vi "Initialize.vi"(8 "error in (no error)":errorcluster, 11 "UDP Thread UI in":refnum<class "UDP Thread User Interface.lvclass">) -> (0 "error out":errorcluster, 3 "UDP Thread UI out":refnum<class "UDP Thread User Interface.lvclass">)   [LabVIEW 2017, in "DSF Core.lvlib" / "UDP Thread User Interface.lvclass"]
uses:
  UDP Thread User Interface.lvclass
  C:/Git/DSF/Core/Classes/User Interface/User Interface.lvclass
  Configuration/UDP Thread Configuration.lvclass
  C:/Git/DSF/Core/Classes/Configuration/Configuration.lvclass
  Classes/User Interface/User Interface.lvclass
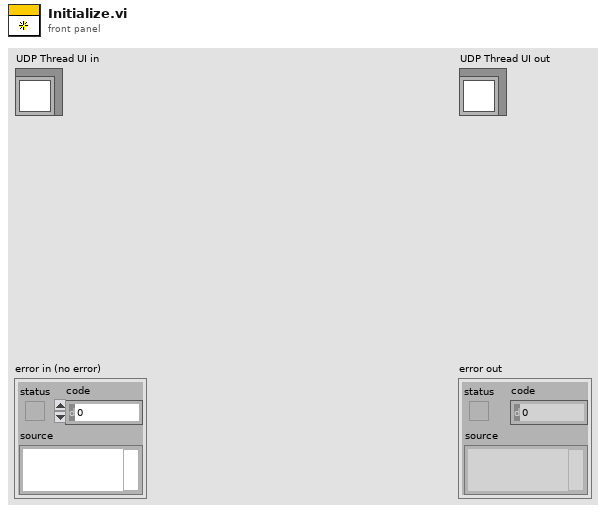
[diagram p1: front panel]
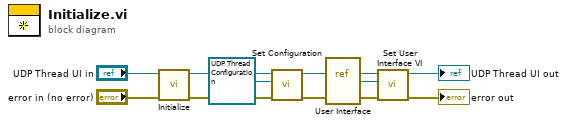
[diagram p0: block diagram]
diagram:
  n1 = call-parent "Initialize.vi"("error in (no error)"="error in (no error)", "User Interface in"="UDP Thread UI in") -> ("error out"=w7:errorcluster, "User Interface out"=w8:refnum<class "UDP Thread User Interface.lvclass">)  [unwired: 8 in]
  n2 = call "Set Configuration.vi"("error in (no error)"=w7, "configuration"=refnum<class "UDP Thread Configuration.lvclass"> refnum ("DSF Core.lvlib:DSF UDP Thread Configuration"), "User Interface in"=w8) -> ("error out"=w6:errorcluster, "User Interface out"=w5:refnum<class "UDP Thread User Interface.lvclass">)  [unwired: 7 in]
  n3 = vi-ref "User Interface.vi"() -> (w2:refnum<vi>)
  n4 = call "Set User Interface VI.vi"("error in (no error)"=w6, "vi"=w2, "User Interface in"=w5) -> ("error out"=→"error out":errorcluster, "User Interface out"=→"UDP Thread UI out":refnum<class "UDP Thread User Interface.lvclass">)  [unwired: 7 in]
